vi "Read LAYER.vi"(8 "error in (no error)":errorcluster, 11 "Geometric in":refnum<class "Geometric.lvclass">) -> (0 "error out":errorcluster, 2 "LAYER":i16, 3 "Geometric out":refnum<class "Geometric.lvclass">)   [LabVIEW 2019, in "Geometric.lvclass"]
uses:
  Geometric.lvclass
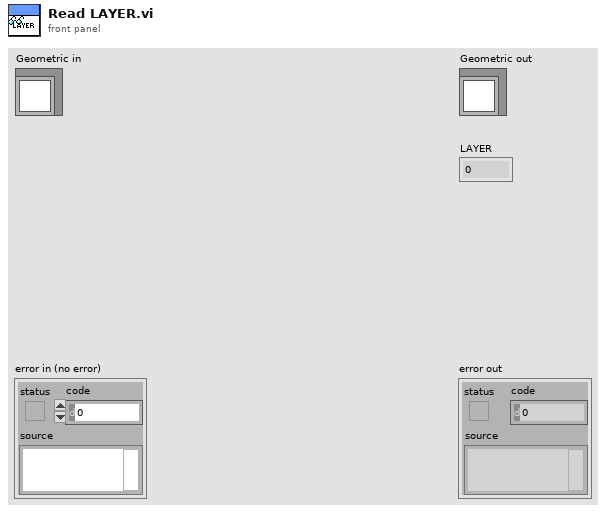
[diagram p1: front panel]
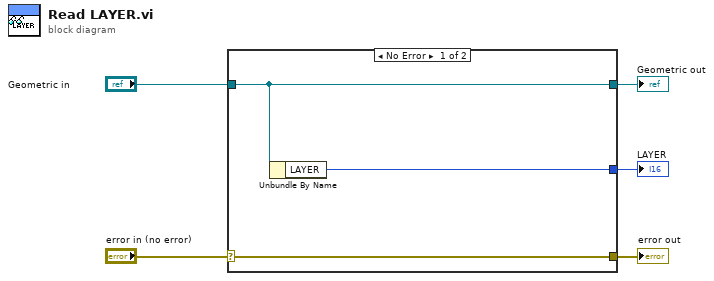
[diagram p0: block diagram]
diagram:
  n1 = case shown="No Error" "error in (no error)" {
    selector: "error in (no error)" -> [w8 w9]
    tunnel: [w8 w9] -> w4
    tunnel: [w7 w10] -> w2
    tunnel: "Geometric in" -> [w7 w10]
    tunnel: [w6 _] -> w1
    frame No Error {
      n2 = Unbundle By Name(w7) -> ("LAYER"=w6:i16)
    }
    frame Error {
    }
  }
  "error out" <- w4
  "Geometric out" <- w2
  "LAYER" <- w1
